vi "TCP Close.vi"(2 "error in (no error)":errorcluster, 3 "connection ID":refnum<k5>) -> ()   [LabVIEW 2018]
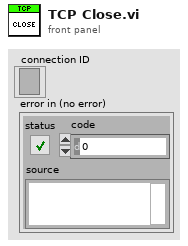
[diagram p1: front panel]
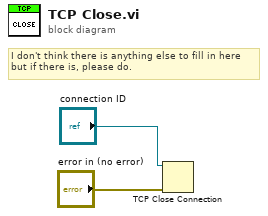
[diagram p0: block diagram]
diagram:
  # "I don't think there is anything else to fill in here\nbut if there is, please do."
  n1 = TCP Close Connection(connection ID="connection ID", error in (no error)="error in (no error)") -> ()  [unwired: 1 in, 2 out]
